vi "WriteChannels_MultipleValues.vi"(4 "Values":bool[](array[boolean]), 5 "Channels":i32[](array[numeric]), 6 "error in":errorcluster) -> (0 "error out":errorcluster)   [LabVIEW 2014, in "GPIO.lvlib"]
doc: "Writes values to the correesponding channels. All channels must be configured as an output before calling this VI."
uses:
  GPIO.lvlib
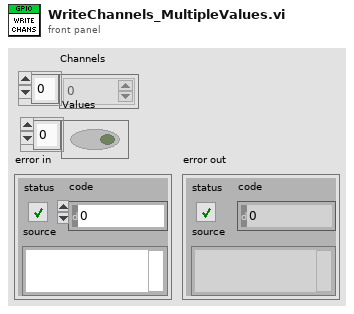
[diagram p1: front panel]
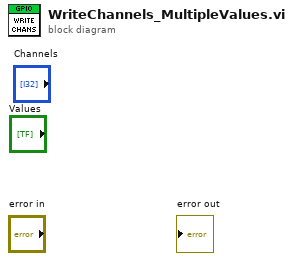
[diagram p0: block diagram]
diagram:
